vi "IsItemInPrivateScope.vi"(8 "error in (no error)":errorcluster, 10 "Item":refnum<vi>) -> (0 "error out":errorcluster, 2 "Is Private?":bool)   [LabVIEW 2017, in "Whitelist.lvclass"]
uses:
  Whitelist.lvclass
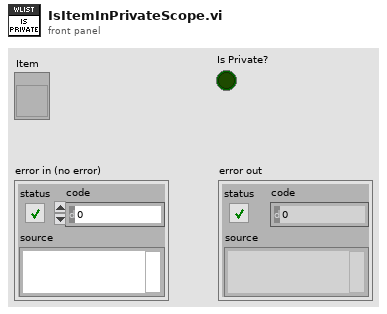
[diagram p1: front panel]
types:
  T1 = enum32{"invalid scope", "public", "private", "protected", "community"}
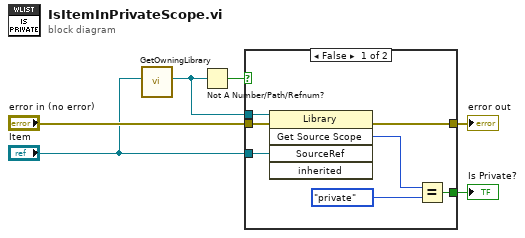
[diagram p0: block diagram]
diagram:
  n1 = call "GetOwningLibrary.vi"("Parent"="Item") -> ("Owner"=w2:refnum<vi>)  [unwired: 10 in]
  n2 = Not A Number/Path/Refnum?(number/path/refnum=w2) -> (NaN/Path/Refnum?=w1:bool)
  n3 = case shown="False" w1 {
    tunnel: "error in (no error)" -> [w13 w14]
    tunnel: [w12 w14] -> w5
    tunnel: [w11 _] -> w4
    tunnel: "Item" -> [w8 _]
    tunnel: w2 -> [w7 _]
    frame False {
      n4 = invoke class="Library" method="Get Source Scope"(reference=w7, error in=w13, "SourceRef"=w8) -> (error out=w12:errorcluster, "GetSourceScope"=w10:T1)  [unwired: 2 in, 3 out]
      n5 = Equal?(x=w10, y=T1."private") -> (x = y?=w11:bool)
    }
    frame True {
    }
  }
  "error out" <- w5
  "Is Private?" <- w4
